vi "ADC_Off_Gain_compute.vi"(7 "VREF_Measured":dbl=2.5 format="%#_13g", 10 "Voltage_Array":dbl[](array[numeric]) format="%#_8g", 11 "Code":dbl[](array[numeric]) format="%#_8g") -> (0 "Gain":dbl, 1 "Gain_Error_(LSB)":dbl, 2 "Offset_Error":dbl, 3 "slope":dbl)   [LabVIEW 2019]
uses:
  <vilib>/Analysis/6fits.llb/Curve Fitting Criteria.ctl
  <vilib>/Analysis/NI_AALPro.lvlib
panel:
  in  "ADC Bits":i32=12
  out "Y":dbl
  out "Meas_Code":dbl
  out "Plot":cluster{dbl[], dbl[]}(graph)
  out "1/x":dbl format="%#_6p"
  out "Plots 3":cluster{dbl[], dbl[]}(graph)
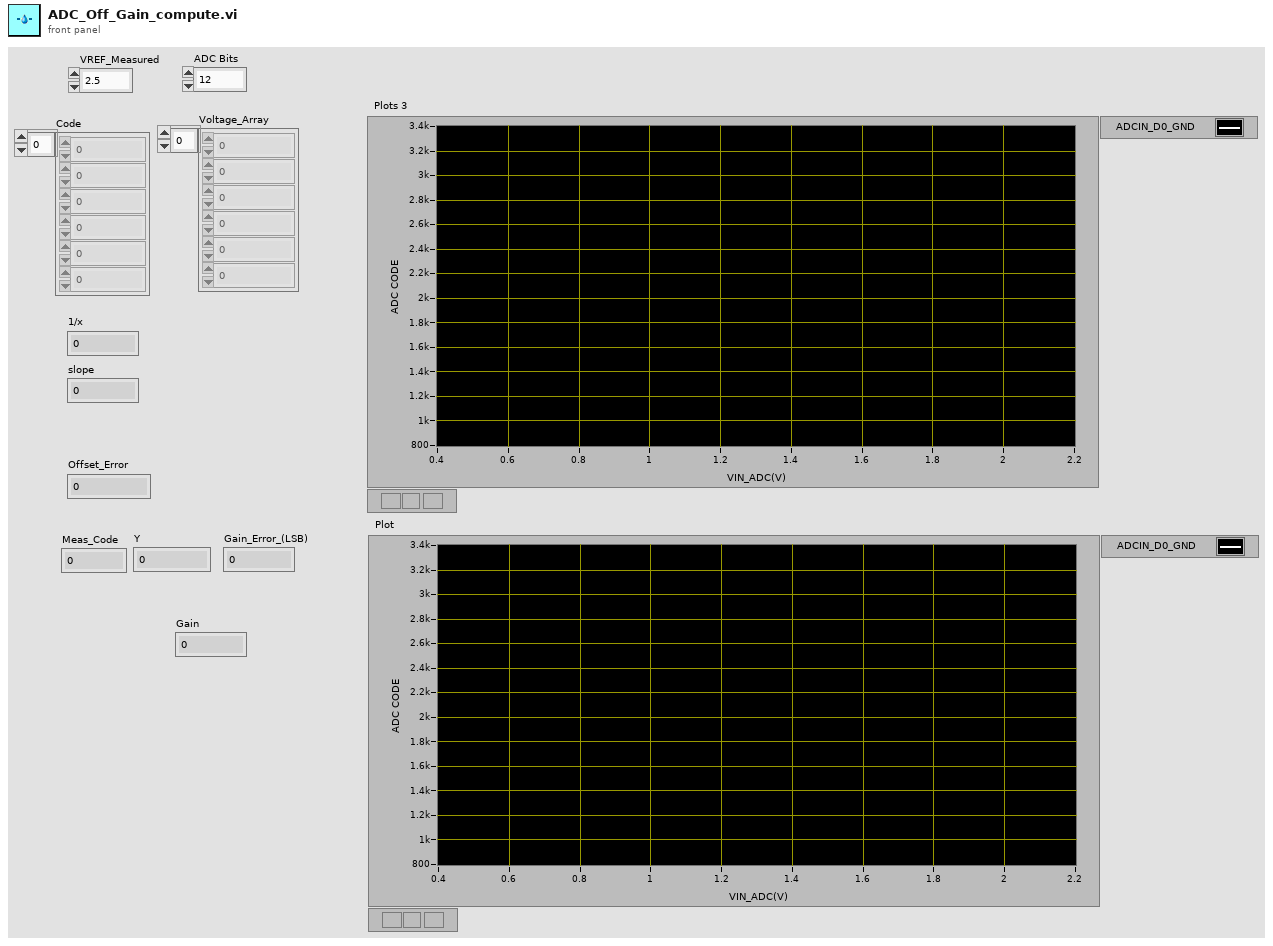
[diagram p1: front panel]
types:
  T1 = typedef "NI_AALPro.lvlib/Curve Fitting Criteria.ctl" = u16
  T2 = cluster{"Voltage_Array":dbl[], "Best Linear Fit":dbl[]}
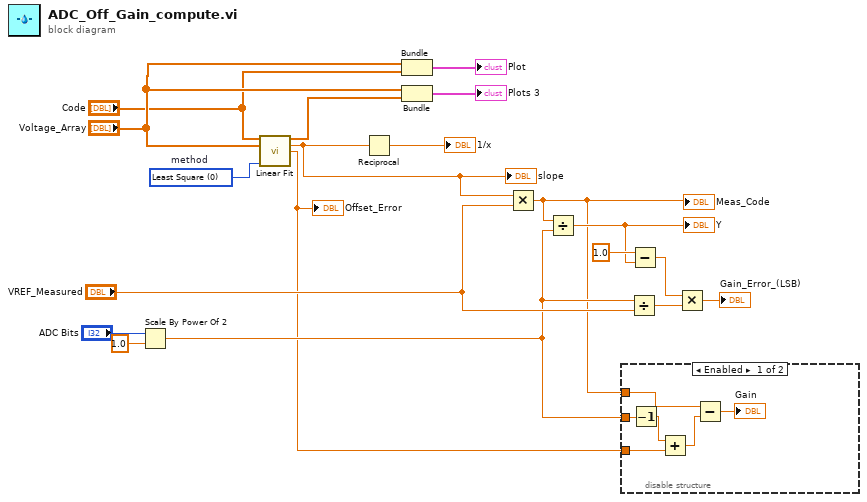
[diagram p0: block diagram]
diagram:
  w19 = T1 0 items=["Least Square", "Least Absolute Residual", "Bisquare"]  # method
  n1 = Scale By Power Of 2(n="ADC Bits", x=1.0) -> (x*2^n=w5:dbl)
  n2 = call <vilib>:"Linear Fit.vi"("Y"="Code", "X"="Voltage_Array", "method"=w19) -> ("Best Linear Fit"=w14:dbl[], "slope"=w15:dbl, "intercept"=w3:dbl)  [unwired: 8 in, 2 out]
  "slope" <- w15
  "Offset_Error" <- w3
  n3 = Reciprocal(x=w15) -> (1/x=→"1/x":dbl)
  n4 = Bundle("Voltage_Array"="Voltage_Array", "Code"="Code") -> (→"Plot":cluster{"Voltage_Array":dbl[], "Code":dbl[]})  [unwired: 1 in]
  n5 = Bundle("Voltage_Array"="Voltage_Array", "Best Linear Fit"=w14) -> (→"Plots 3":T2)  [unwired: 1 in]
  n6 = Multiply(x=w15, y="VREF_Measured") -> (x*y=w4:dbl)
  "Meas_Code" <- w4
  n7 = Divide(x=w4, y=w5) -> (x/y=w10:dbl)
  "Y" <- w10
  n8 = disable-structure shown="Enabled" {
    disable-tunnel: w5 -> [w25 _]
    disable-tunnel: w4 -> [w24 _]
    disable-tunnel: w3 -> [w20 _]
    frame Enabled {
      n9 = Decrement(x=w25) -> (x-1=w21:dbl)
      n10 = Add(x=w21, y=w20) -> (x+y=w22:dbl)
      n11 = Subtract(x=w24, y=w22) -> (x-y=→"Gain":dbl)
    }
    frame Disabled {
    }
  }
  n12 = Divide(x=w5, y="VREF_Measured") -> (x/y=w8:dbl)
  n13 = Subtract(x=1.0, y=w10) -> (x-y=w9:dbl)
  n14 = Multiply(x=w9, y=w8) -> (x*y=→"Gain_Error_(LSB)":dbl)
